vi "Get Current.vi"(8 "error in (no error)":errorcluster, 11 "KUKA youBot arm motor_EtherCAT in":refnum<class "NI_Robotics_KUKA youBot Arm Motor_EtherCAT.lvclass">) -> (0 "error out":errorcluster, 2 "current (A)":dbl, 3 "KUKA youBot arm motor_EtherCAT out":refnum<class "NI_Robotics_KUKA youBot Arm Motor_EtherCAT.lvclass">)   [LabVIEW 2017, in "NI_Robotics_KUKA youBot Host.lvlib" / "NI_Robotics_KUKA youBot Arm Motor_EtherCAT.lvclass"]
uses:
  <vilib>/robotics/KUKA youBot/Motor/Arm Motor EtherCAT/NI_Robotics_KUKA youBot Arm Motor_EtherCAT.lvclass
  <vilib>/robotics/KUKA youBot/Motor/Arm Motor EtherCAT/NI_Robotics_KUKA youBot Arm Motor_EtherCAT.lvclass/NI_Robotics_KUKA youBot Arm Motor_EtherCAT.ctl
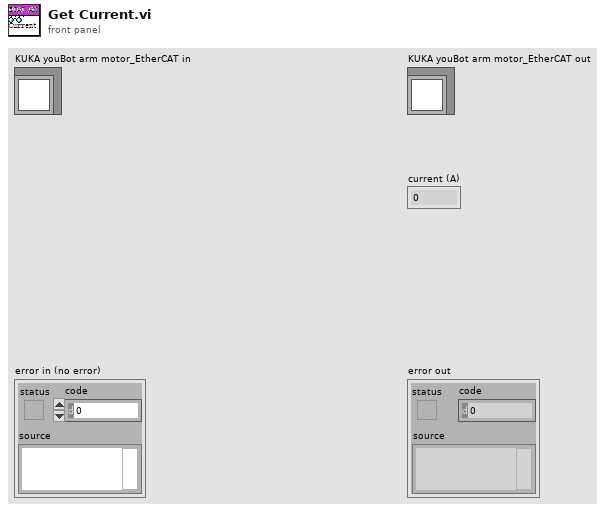
[diagram p1: front panel]
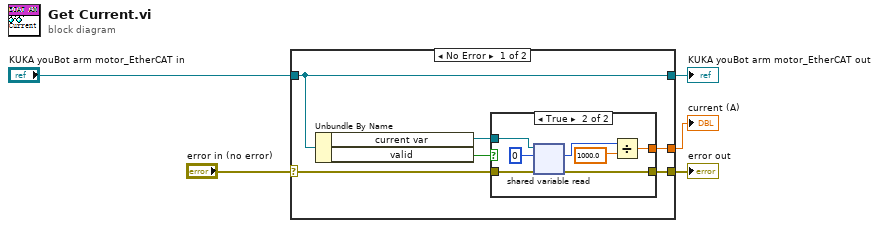
[diagram p0: block diagram]
diagram:
  n1 = case shown="No Error" "error in (no error)" {
    selector: "error in (no error)" -> [w8 w20]
    tunnel: [w6 w20] -> w4
    tunnel: [w11 w21] -> w2
    tunnel: "KUKA youBot arm motor_EtherCAT in" -> [w11 w21]
    tunnel: [w7 _] -> w1
    frame No Error {
      n2 = Unbundle By Name(w11) -> ("current var"=w9:refnum<k21>, "valid"=w10:bool)
      n3 = case shown="True" w10 {
        tunnel: w9 -> [_ w19]
        tunnel: w8 -> [w12 w17]
        tunnel: [_ w14] -> w7
        tunnel: [w12 w13] -> w6
        frame False {
        }
        frame True {
          n4 = shared-variable-read(w19, w17, 0 ("data type")) -> (w13:errorcluster, w16:i32)  [unwired: 2 out]
          n5 = Divide(x=w16, y=1000.0) -> (x/y=w14:dbl)
        }
      }
    }
    frame Error {
    }
  }
  "error out" <- w4
  "KUKA youBot arm motor_EtherCAT out" <- w2
  "current (A)" <- w1
